vi "Start placeholder.vi"(11 "TEMPLATE Actor in":refnum<class "TEMPLATE Actor.lvclass">) -> (0 "Error out":errorcluster, 3 "TEMPLATE Actor out":refnum<class "TEMPLATE Actor.lvclass">)   [LabVIEW 2025, in "_Template.lvlib" / "Templates.lvlib" / "TEMPLATE Actor.lvlib" / "TEMPLATE Actor.lvclass"]
uses:
  TEMPLATE Actor.lvclass
  TEMPLATE Actor.lvclass/TEMPLATE Actor.ctl
  C:/git/jettl/src/jettl Tools/_Template/Templates/TEMPLATE Actor/TEMPLATE Actor/TEMPLATE Actor.lvclass
  C:/git/jettl/src/jettl/jettl/Actor/Actor/Actor.lvclass
  C:/git/jettl/src/jettl/jettl/Finish Msg/Finish/Finish.lvclass
  jettl/jettl/Actor/Actor.lvlib
  Aliases For Created.ctl
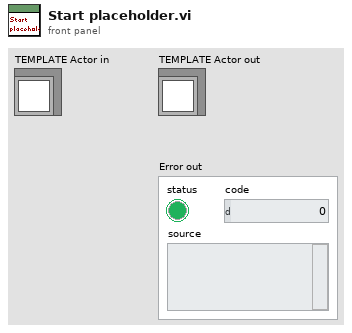
[diagram p1: front panel]
types:
  T1 = typedef "_Template.lvlib/Templates.lvlib/TEMPLATE Actor.lvlib/TEMPLATE Actor.lvclass/Aliases For Created.ctl" = enum16{""}
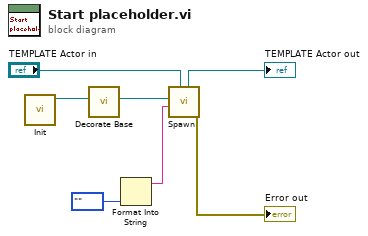
[diagram p0: block diagram]
diagram:
  n1 = call "Init.vi"() -> ("TEMPLATE Actor out"=w2:refnum<class "TEMPLATE Actor.lvclass">)  [unwired: 11 in]
  n2 = call "Decorate Base.vi"("Actor To Decorate Base"=w2) -> ("Decorated Base Actor"=w1:refnum<class "TEMPLATE Actor.lvclass">)  [unwired: 10 in]
  n3 = Format Into String(Aliases_For_Created."" ("Aliases For Created")) -> (resulting string=w4:string)  [unwired: 3 in, 1 out]
  n4 = call "Spawn.vi"("Actor in"="TEMPLATE Actor in", "UID"=w4, "Actor"=w1) -> ("Error out"=→"Error out":errorcluster, "Actor out"=→"TEMPLATE Actor out":refnum<class "TEMPLATE Actor.lvclass">)  [unwired: 7 in]
